vi "OrientationFSM.vi"(8 "Rubik's Moves":T1) -> (3 "Final Orientation":T2)   [LabVIEW 2017]
uses:
  Projekt-RubikLibrary/OrientationState.ctl
  Projekt-RubikLibrary/RubikMoves.ctl
  Projekt-RubikLibrary/RubikLibrary.lvlib
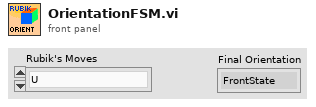
[diagram p1: front panel]
types:
  T1 = typedef "RubikLibrary.lvlib/RubikMoves.ctl" = enum16{"U", "U'", "F", "F'", "D", "D'", "B", "B'", "L", "L'", "R", "R'"}
  T2 = typedef "RubikLibrary.lvlib/OrientationState.ctl" = enum16{"FrontState", "UpState", "BackState", "DownState"}
  T3 = typedef "RubikLibrary.lvlib/RubikOps.ctl" = cluster{"Device":enum16{"Servo", "SyncTurn", "Grip"}, "Angles":T4[], "Grips":bool[]}
  T4 = typedef "RubikLibrary.lvlib/ServoAbsAngleControl.ctl" = enum16{"+90°", "0°", "-90°"}
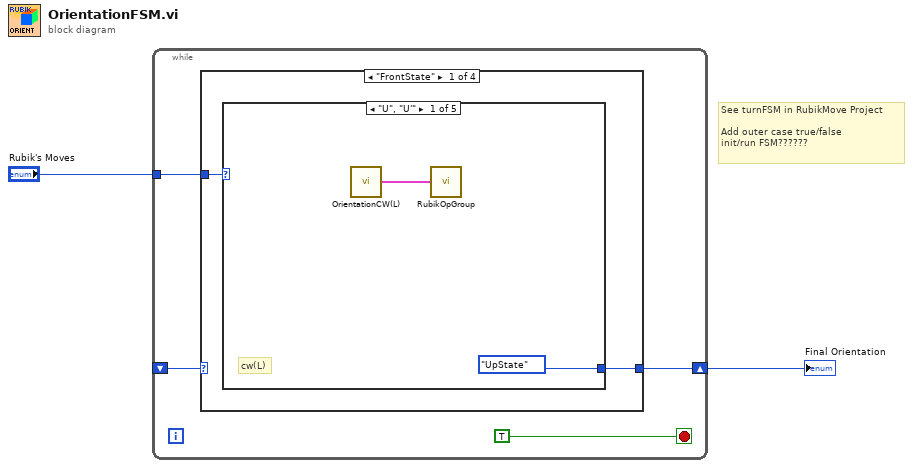
[diagram p0: block diagram]
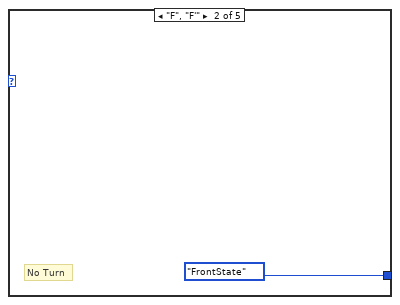
[diagram p2: hidden frame]
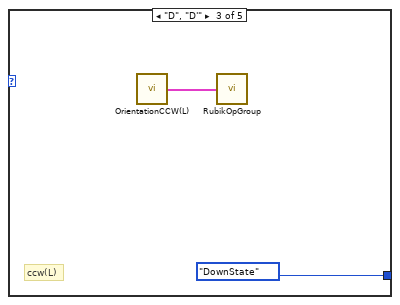
[diagram p3: hidden frame]
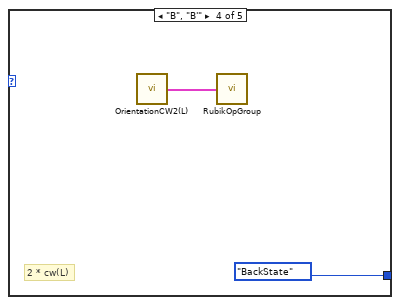
[diagram p4: hidden frame]
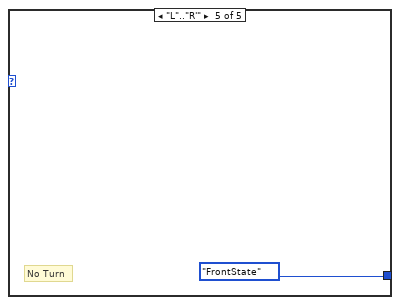
[diagram p5: hidden frame]
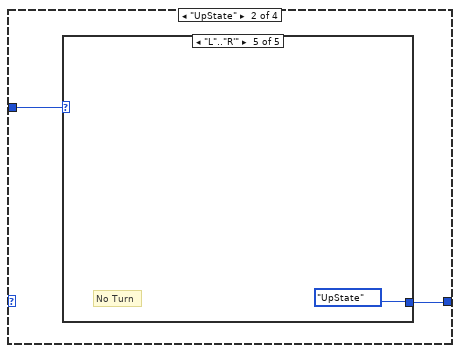
[diagram p6: hidden frame]
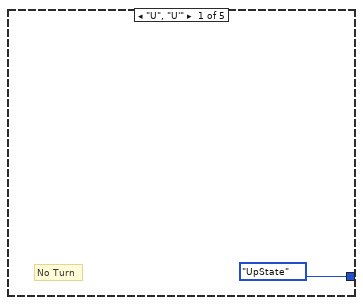
[diagram p7: hidden frame]
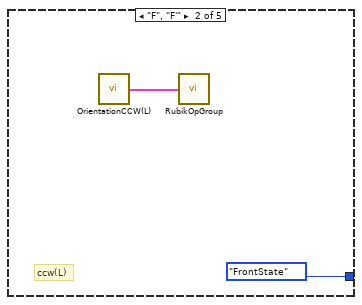
[diagram p8: hidden frame]
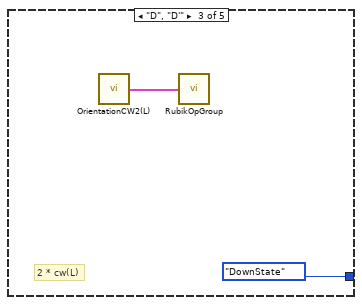
[diagram p9: hidden frame]
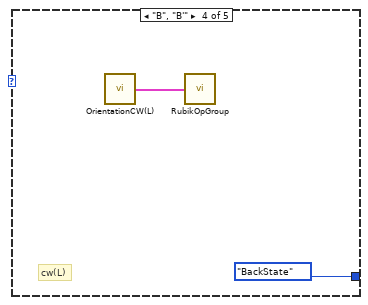
[diagram p10: hidden frame]
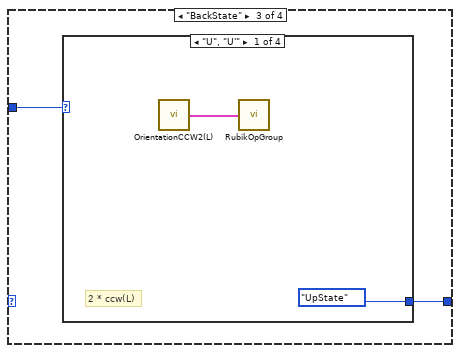
[diagram p11: hidden frame]
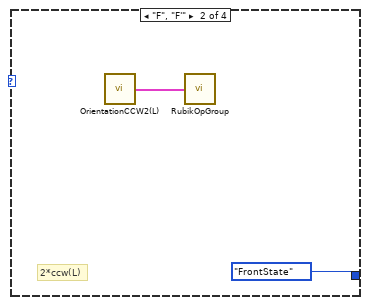
[diagram p12: hidden frame]
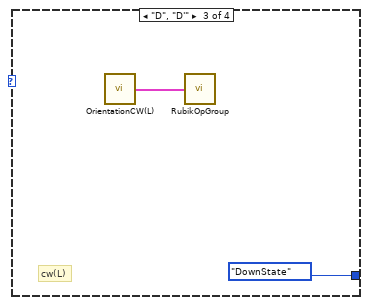
[diagram p13: hidden frame]
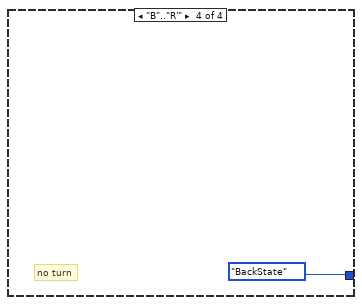
[diagram p14: hidden frame]
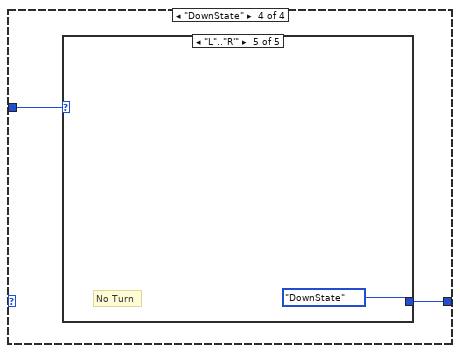
[diagram p15: hidden frame]
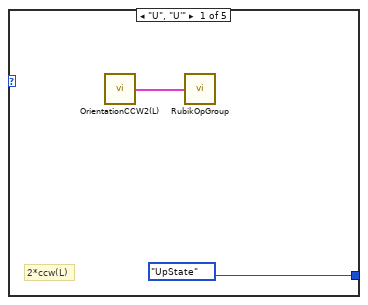
[diagram p16: hidden frame]
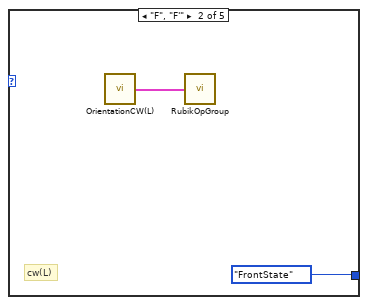
[diagram p17: hidden frame]
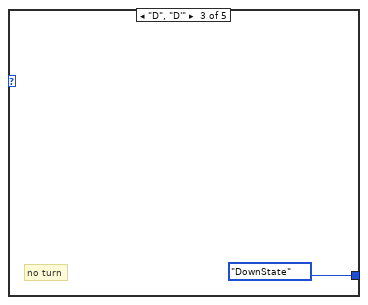
[diagram p18: hidden frame]
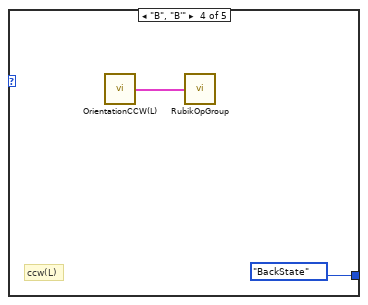
[diagram p19: hidden frame]
diagram:
  # "See turnFSM in RubikMove Project\n\nAdd outer case true/false\ninit/run FSM??????"
  n1 = while {
    tunnel: "Rubik's Moves" -> [w6]
    shift-right: [w3] -> w2
    shift-left: _ -> [w4]
    stop <- TRUE stop-if-true
    n2 = case shown="\"FrontState\"" w4 {
      tunnel: w6 -> [w8 w18 w28 w36]
      tunnel: [w7 w17 w27 w37] -> w3
      frame "FrontState" {
        n3 = case shown="\"U\", \"U'\"" w8 {
          tunnel: [OrientationState."UpState" ("Initial Orientation") OrientationState."FrontState" ("Initial Orientation") OrientationState."DownState" ("Initial Orientation") OrientationState."BackState" ("Initial Orientation") OrientationState."FrontState" ("Initial Orientation")] -> w7
          frame "U", "U'" {
            # "cw(L)"
            n4 = call "OrientationCW(L).vi"() -> ("Array of Operations (out)"=w9:T3[])  [unwired: 2 in]
            n5 = call "RubikOpGroup.vi"("Array of Operations"=w9) -> ()  [unwired: 2 in, 1 out]
          }
          frame "F", "F'" {
            # "No Turn"
          }
          frame "D", "D'" {
            # "ccw(L)"
            n6 = call "OrientationCCW(L).vi"() -> ("Array of Operations (out)"=w12:T3[])  [unwired: 2 in]
            n7 = call "RubikOpGroup.vi"("Array of Operations"=w12) -> ()  [unwired: 2 in, 1 out]
          }
          frame "B", "B'" {
            # "2 * cw(L)"
            n8 = call "OrientationCW2(L).vi"() -> ("Array of Operations (out)"=w14:T3[])  [unwired: 2 in]
            n9 = call "RubikOpGroup.vi"("Array of Operations"=w14) -> ()  [unwired: 2 in, 1 out]
          }
          frame "L".."R'" {
            # "No Turn"
          }
        }
      }
      frame "UpState" {
        n10 = case shown="\"L\"..\"R'\"" w18 {
          tunnel: [OrientationState."UpState" ("Initial Orientation") OrientationState."FrontState" ("Initial Orientation") OrientationState."DownState" ("Initial Orientation") OrientationState."BackState" ("Initial Orientation") OrientationState."UpState" ("Initial Orientation")] -> w17
          frame "U", "U'" {
            # "No Turn"
          }
          frame "F", "F'" {
            # "ccw(L)"
            n11 = call "OrientationCCW(L).vi"() -> ("Array of Operations (out)"=w20:T3[])  [unwired: 2 in]
            n12 = call "RubikOpGroup.vi"("Array of Operations"=w20) -> ()  [unwired: 2 in, 1 out]
          }
          frame "D", "D'" {
            # "2 * cw(L)"
            n13 = call "OrientationCW2(L).vi"() -> ("Array of Operations (out)"=w22:T3[])  [unwired: 2 in]
            n14 = call "RubikOpGroup.vi"("Array of Operations"=w22) -> ()  [unwired: 2 in, 1 out]
          }
          frame "B", "B'" {
            # "cw(L)"
            n15 = call "OrientationCW(L).vi"() -> ("Array of Operations (out)"=w24:T3[])  [unwired: 2 in]
            n16 = call "RubikOpGroup.vi"("Array of Operations"=w24) -> ()  [unwired: 2 in, 1 out]
          }
          frame "L".."R'" {
            # "No Turn"
          }
        }
      }
      frame "BackState" {
        n17 = case shown="\"U\", \"U'\"" w28 {
          tunnel: [OrientationState."UpState" ("Initial Orientation") OrientationState."FrontState" ("Initial Orientation") OrientationState."DownState" ("Initial Orientation") OrientationState."BackState" ("Initial Orientation")] -> w27
          frame "U", "U'" {
            # "2 * ccw(L)"
            n18 = call "OrientationCCW2(L).vi"() -> ("Array of Operations (out)"=w29:T3[])  [unwired: 2 in]
            n19 = call "RubikOpGroup.vi"("Array of Operations"=w29) -> ()  [unwired: 2 in, 1 out]
          }
          frame "F", "F'" {
            # "2*ccw(L)"
            n20 = call "OrientationCCW2(L).vi"() -> ("Array of Operations (out)"=w31:T3[])  [unwired: 2 in]
            n21 = call "RubikOpGroup.vi"("Array of Operations"=w31) -> ()  [unwired: 2 in, 1 out]
          }
          frame "D", "D'" {
            # "cw(L)"
            n22 = call "OrientationCW(L).vi"() -> ("Array of Operations (out)"=w33:T3[])  [unwired: 2 in]
            n23 = call "RubikOpGroup.vi"("Array of Operations"=w33) -> ()  [unwired: 2 in, 1 out]
          }
          frame "B".."R'" {
            # "no turn"
          }
        }
      }
      frame "DownState" {
        n24 = case shown="\"L\"..\"R'\"" w36 {
          tunnel: [OrientationState."UpState" ("Initial Orientation") OrientationState."FrontState" ("Initial Orientation") OrientationState."DownState" ("Initial Orientation") OrientationState."BackState" ("Initial Orientation") OrientationState."DownState" ("Initial Orientation")] -> w37
          frame "U", "U'" {
            # "2*ccw(L)"
            n25 = call "OrientationCCW2(L).vi"() -> ("Array of Operations (out)"=w38:T3[])  [unwired: 2 in]
            n26 = call "RubikOpGroup.vi"("Array of Operations"=w38) -> ()  [unwired: 2 in, 1 out]
          }
          frame "F", "F'" {
            # "cw(L)"
            n27 = call "OrientationCW(L).vi"() -> ("Array of Operations (out)"=w40:T3[])  [unwired: 2 in]
            n28 = call "RubikOpGroup.vi"("Array of Operations"=w40) -> ()  [unwired: 2 in, 1 out]
          }
          frame "D", "D'" {
            # "no turn"
          }
          frame "B", "B'" {
            # "ccw(L)"
            n29 = call "OrientationCCW(L).vi"() -> ("Array of Operations (out)"=w43:T3[])  [unwired: 2 in]
            n30 = call "RubikOpGroup.vi"("Array of Operations"=w43) -> ()  [unwired: 2 in, 1 out]
          }
          frame "L".."R'" {
            # "No Turn"
          }
        }
      }
    }
  }
  "Final Orientation" <- w2
